vi "Data Unsubscribed.vi"(8 "error in (no error)":errorcluster, 10 "Groups":string[](array[string]), 11 "Group Data Handler in":refnum<class "Group Data Handler.lvclass">) -> (0 "error out":errorcluster, 3 "Group Data Handler out":refnum<class "Group Data Handler.lvclass">)   [LabVIEW 2020, in "VolatusHistorian.lvlib" / "Group Data Handler.lvclass"]
uses:
  Group Data Handler.lvclass
  Group Data Handler.lvclass/Group Data Handler.ctl
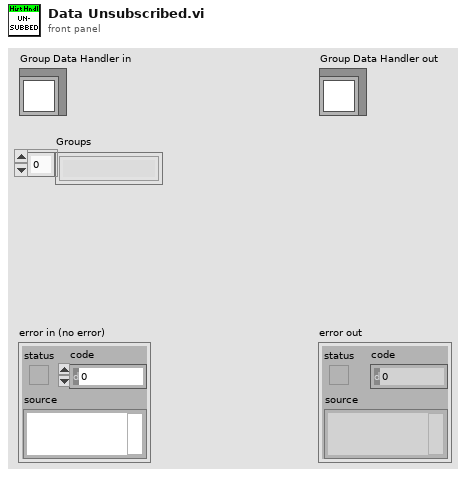
[diagram p1: front panel]
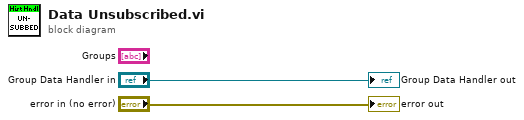
[diagram p0: block diagram]
diagram:
  "error out" <- "error in (no error)"
  "Group Data Handler out" <- "Group Data Handler in"
